vi "RF Rec DDC (Two Channels).vi"(0 "data in":T1[](array[typedef]), 1 "reset":bool, 5 "start trigger":bool, 9 "enable":bool[](array[boolean]), 11 "ddc parameters":T2[](array[typedef]) {"frequency shift" format="%#.48g"}) -> (4 "data out":u32[](array[numeric]), 6 "number of overflows":u64[](array[numeric]), 10 "output valid":bool, 14 "dsp reset done":bool)   [LabVIEW 2018]
doc: "Digital downconverter (DDC). Implemented with FPGA-based DSP.\n\n<B>Input Parameters</B>\n\n<B>data in</B> is the I and Q data to be downconverted along with overflow information.\n\n<B>start trigger</B> triggers the Rx signal chain if an Rx stream is enabled.\n\n<B>enable</B> specifies which streams are enabled.\n\n<B>ddc parameters</B> are the downconversion parameters utilized by the DSP chain.\n\n<B>reset</B> the DSP downconversion signal chain.\n\n<B>Output Parameters</B>\n\n<B>dsp reset done</B> indicates that the DSP downconversion signal chain completed reset.\n\n<B>data out</B> is the downconverted data.\n\n<B>number of overflows</B> is the number of times the DSP chain overflowed on fixed point conversion of 'data in'.\n\n<B>output valid</B> specifies when 'data out' is valid."
uses:
  RF Rec DDC Parameters.ctl
  <instrlib>/_niInstr/DSP/v1/Shared/Public/IQ Impairments.ctl
  <instrlib>/_niInstr/DSP/v1/Shared/Public/IQ Data.ctl
  <instrlib>/_niInstr/DSP/v1/Shared/niInstr DSP v1 Shared.lvlib
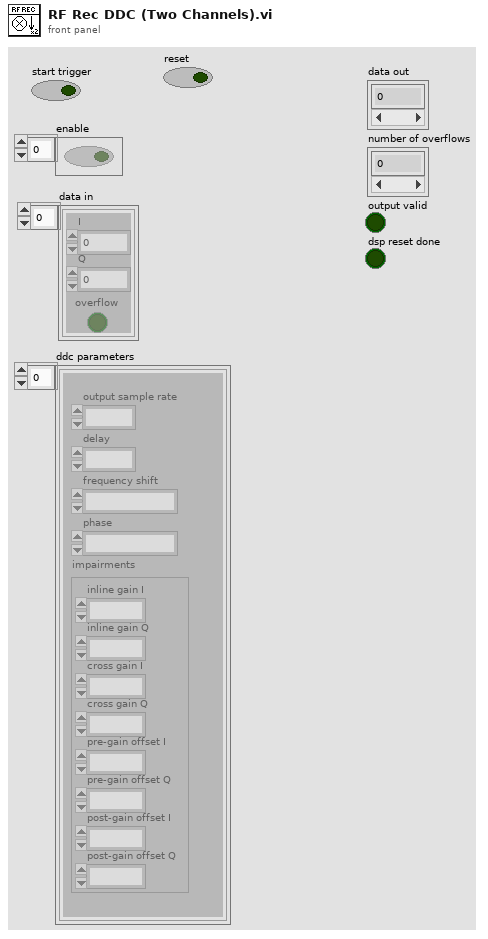
[diagram p1: front panel]
types:
  T1 = typedef "niInstr DSP v1 Shared.lvlib/IQ Data.ctl" = cluster{"I":fxp<+/-,18,1>, "Q":fxp<+/-,18,1>, "overflow":bool}
  T2 = typedef "RF Rec DDC Parameters.ctl" = cluster{"output sample rate":fxp<+,48,1>, "delay":fxp<+/-,16,0>, "frequency shift":fxp<+/-,48,0>, "impairments":T3, "phase":fxp<+/-,21,0>}
  T3 = typedef "niInstr DSP v1 Shared.lvlib/IQ Impairments.ctl" = cluster{"inline gain I":fxp<+/-,18,1>, "inline gain Q":fxp<+/-,18,1>, "cross gain I":fxp<+/-,18,1>, "cross gain Q":fxp<+/-,18,1>, "pre-gain offset I":fxp<+/-,18,1>, "pre-gain offset Q":fxp<+/-,18,1>, "post-gain offset I":fxp<+/-,18,1>, "post-gain offset Q":fxp<+/-,18,1>}
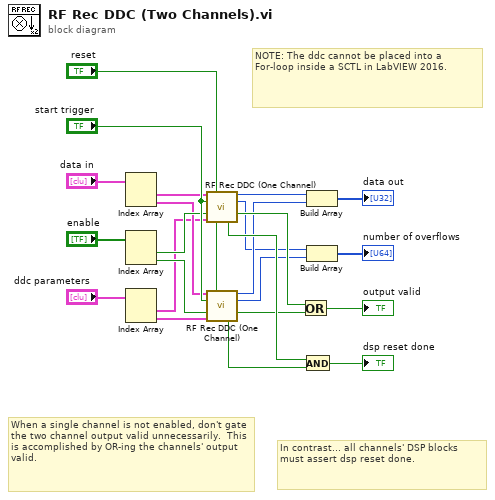
[diagram p0: block diagram]
diagram:
  # "NOTE: The ddc cannot be placed into a For-loop inside a SCTL in LabVIEW 2016."
  # "When a single channel is not enabled, don't gate the two channel output valid unnecessarily.  This is accomplished by OR-ing the channels' output valid."
  # "In contrast... all channels' DSP blocks must assert dsp reset done."
  n1 = Index Array(array="data in") -> (element #1=w7:T1, element #2=w3:T1)  [unwired: 2 in]
  n2 = Index Array(array="enable") -> (element #1=w5:bool, element #2=w4:bool)  [unwired: 2 in]
  n3 = Index Array(array="ddc parameters") -> (element #1=w2:T2, element #2=w6:T2)  [unwired: 2 in]
  n4 = call "RF Rec DDC (One Channel).vi"("data in"=w7, "reset"="reset", "start trigger"="start trigger", "enable"=w5, "ddc parameters"=w2) -> ("data out"=w16:u32, "number of overflows"=w13:u64, "output valid"=w18:bool, "dsp reset done"=w19:bool)  [unwired: 7 in]
  n5 = call "RF Rec DDC (One Channel).vi"("data in"=w3, "reset"="reset", "start trigger"="start trigger", "enable"=w4, "ddc parameters"=w6) -> ("data out"=w14:u32, "number of overflows"=w12:u64, "output valid"=w17:bool, "dsp reset done"=w20:bool)  [unwired: 7 in]
  n6 = Or(x=w18, y=w17) -> (x .or. y?=→"output valid":bool)
  n7 = And(x=w19, y=w20) -> (x .and. y?=→"dsp reset done":bool)
  n8 = Build Array(w16, w14) -> (→"data out":u32[])
  n9 = Build Array(w13, w12) -> (→"number of overflows":u64[])
